vi "ServerLauncher.vi"   [LabVIEW 2021]
uses:
  Server/Server/Server.lvclass
  C:/Program Files/National Instruments/LabVIEW 2021/vi.lib/ActorFramework/Actor/Actor.lvclass
  <vilib>/ActorFramework/Actor/Actor.lvclass
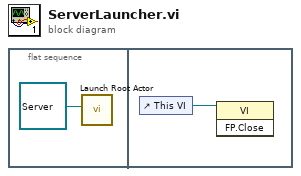
[diagram p0: block diagram]
diagram:
  n1 = flat-sequence {
    frame #0 {
      n2 = call <vilib>:"Launch Root Actor.vi"("Actor"=refnum<class "Server.lvclass"> refnum ("Server.lvlib:Server.lvclass")) -> ()  [unwired: 9 in, 2 out]
    }
    frame #1 {
      n3 = control-ref of="This VI"() -> (w2:refnum<vi>)
      n4 = invoke class="VI" method="FP.Close"(reference=w2) -> ()  [unwired: 2 in, 3 out]
    }
  }
